vi "test1.vi"() -> ()   [LabVIEW 2014]
panel:
  in  "Time Delay in Sec":dbl=1.0
  out "XY Graph":cluster{"Y":dbl[], "Y":dbl[]}[](graph)=[{"Y"=[0.0, 0.0, 1.0, 2.0, 3.0], "Y"=[0.0, 0.3619124610612485, 0.5273101920658294, 0.16637594545862644, 0.42799630595870797]}]
  in  "stop":bool
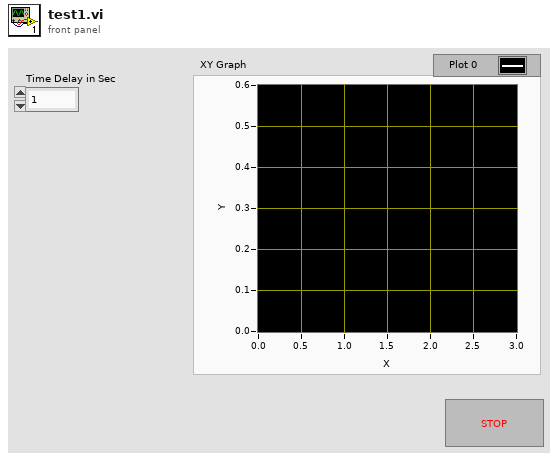
[diagram p1: front panel]
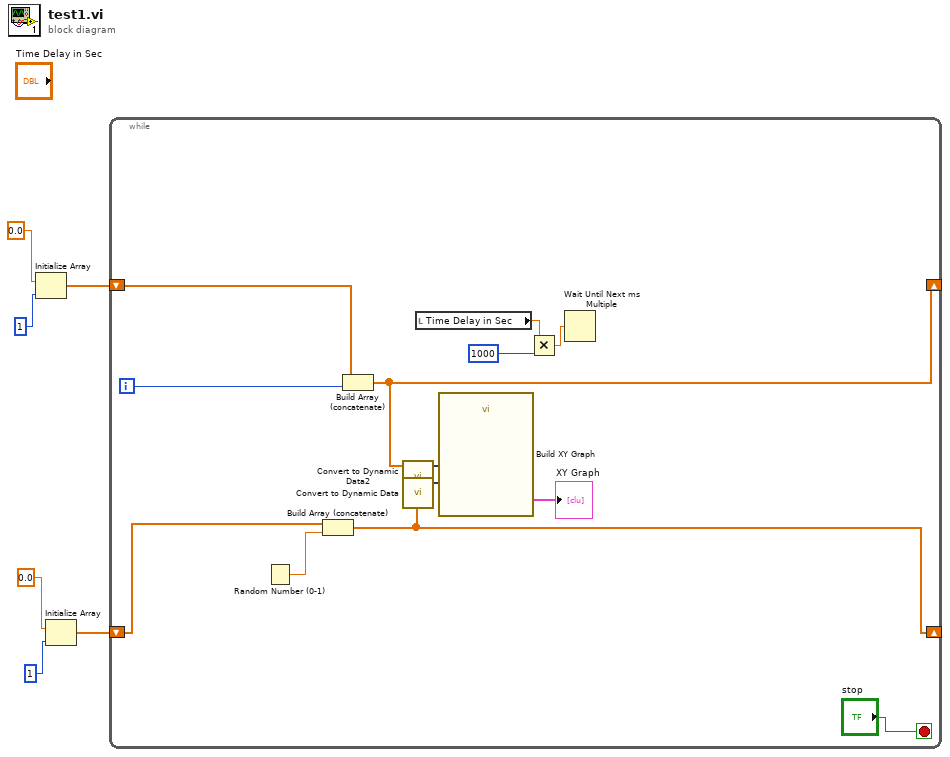
[diagram p0: block diagram]
diagram:
  n1 = Initialize Array(0.0 ("element"), 1 ("dimension size")) -> (w5:dbl[])
  n2 = Initialize Array(0.0 ("element"), 1 ("dimension size")) -> (w1:dbl[])
  n3 = while {
    shift-right: [w12] -> _
    shift-left: w5 -> [w17]
    shift-right: [w14] -> _
    shift-left: w1 -> [w16]
    i -> [w10]
    stop <- "stop" stop-if-true
    n4 = Random Number (0-1)() -> (number: 0 to 1=w15:dbl)
    n5 = Build Array (concatenate)(w16, w15) -> (w14:dbl[])
    n6 = Build Array (concatenate)(w17, w10) -> (w12:dbl[])
    n7 = call "Convert to Dynamic Data2"("Array"=w12) -> ("Dynamic Data Type"=w11:dynamicdata)  [unwired: 3 in]
    n8 = call "Convert to Dynamic Data"("Array"=w14) -> ("Dynamic Data Type"=w13:dynamicdata)  [unwired: 3 in]
    n9 = local read "Time Delay in Sec"() -> (w8:dbl)
    n10 = call "Build XY Graph"("Y Input"=w13, "X Input"=w11) -> ("XY Graph"=→"XY Graph":cluster{"X":dbl[], "Y":dbl[]}[])  [unwired: 8 in, 1 out]
    n11 = Multiply(x=w8, y=u32 1000 ("millisecond multiple")) -> (x*y=w7:dbl)
    n12 = Wait Until Next ms Multiple(millisecond multiple=w7) -> ()  [unwired: 1 out]
  }
